vi "barcodescanner.vi"(8 "Color Sensor Port":T1 items=["Port 1", "Port 2", "Port 3", "Port 4"], 9 "Motors":T2=7 items=["Port A", "Port B", "Port C", "Port D"], 10 "digits":i32, 11 "NXT/EV3":T3) -> (1 "decimal conversiom":i32, 3 "NXT/EV3 2":T3)   [LabVIEW 2016]
uses:
  <vilib>/NXT/Subs/LVHSConnector.ctl
  <vilib>/NXT/LegoClasses/BrickReference/BrickReference.lvclass
  <vilib>/NXT/Block Support/NXT_OutputPort.ctl
  <vilib>/NXT/Block Support/NXT_InputPort.ctl
  <vilib>/NXT/Subs/ColorSensorColors.ctl
  <vilib>/NXT/NXTIO Xnodes/NXTIONodeSubVIs/NXTMotorRunDistance.vi
  <vilib>/NXT/Dual Mode Library/Sensors/EV3_Color_Color.vi
  <vilib>/NXT/NXTIO Xnodes/NXTIOXNode/NXTIO.xnode
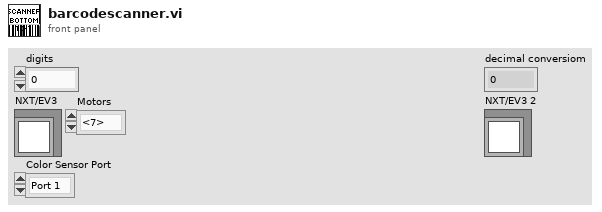
[diagram p1: front panel]
types:
  T1 = typedef "NXT_InputPort.ctl" = u32
  T2 = typedef "NXT_OutputPort.ctl" = u8
  T3 = typedef "LVHSConnector.ctl" = refnum<class "BrickReference.lvclass">
  T4 = typedef "ColorSensorColors.ctl" = enum16{"No Color", "Black", "Blue", "Green", "Yellow", "Red", "White", "Brown"}
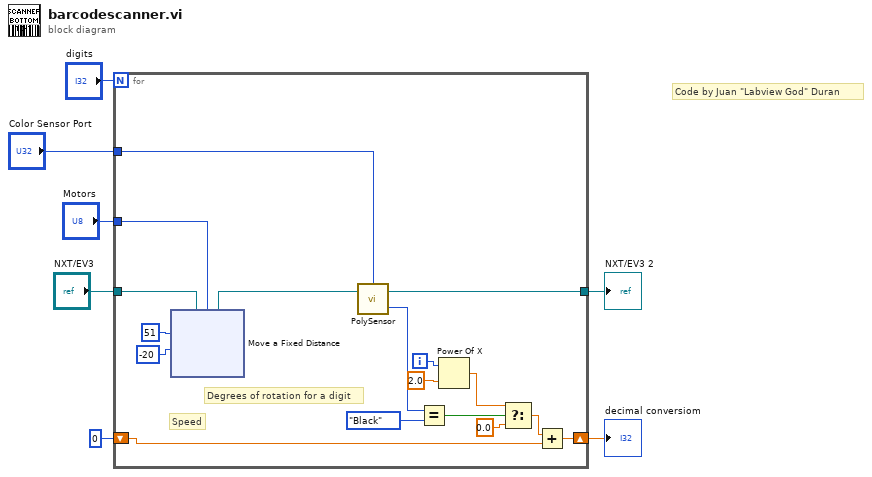
[diagram p0: block diagram]
diagram:
  # "Code by Juan \"Labview God\" Duran"
  n1 = for {
    N: "digits" -> [_]
    shift-right: [w9] -> w5
    shift-left: 0 -> [w10]
    tunnel: "NXT/EV3" -> [w24]
    tunnel: "Motors" -> [w23]
    tunnel: "Color Sensor Port" -> [w19]
    tunnel: [w8] -> w1
    i -> [w15]
    # "Speed"
    # "Degrees of rotation for a digit"
    n2 = xnode "Move a Fixed Distance"("Speed 1"=i8 -20, "Distance 1"=51, "Motors"=w23, "NXT/EV3"=w24) -> ("NXT/EV3"=w20:T3)
    n3 = call-poly <vilib>:"PolySensor.vi"("NXT/EV3"=w20, "Port (Port 1)"=w19) -> ("Detected Color"=w18:T4, "NXT/EV3"=w8:T3)  [unwired: 1 in]
    n4 = Equal?(x=w18, y=ColorSensorColors."Black" ("Detected Color")) -> (x = y?=w14:bool)
    n5 = Power Of X(1:2.0 ("x"), 2:w15) -> (0:w13:dbl)
    n6 = Select(t=w13, s=w14, f=0.0) -> (s? t:f=w11:dbl)
    n7 = Add(x=w11, y=w10) -> (x+y=w9:dbl)
  }
  "decimal conversiom" <- w5
  "NXT/EV3 2" <- w1
